vi "dfd_Lpth Norm Spec Convertion.vi"(8 "error in (no error)":errorcluster, 10 "filter specs":T2[](array[typedef]), 11 "order":i32=21) -> (0 "error out":errorcluster, 2 "band specification":T1 {"magnitude and weight"."frequency point"."weight" format="%.2f"}, 3 "order out":cluster{"# num":i32, "# den":i32}={"# num"=5, "# den"=5})   [LabVIEW 2017, in "NI_DigFilterLicensed.lvlib"]
uses:
  <vilib>/addons/Digital Filter Design/NI_DigFilterLicensed.lvlib
  <vilib>/addons/Digital Filter Design/_LpNorm.llb/dfd_Lp Norm Band Spec.ctl
  <vilib>/addons/Digital Filter Design/_Objects.llb/DFD Filter Specifiction (Design).ctl
panel:
  in  "band specification 2":T1 {"magnitude and weight"."frequency point"."weight" format="%.2f"}
  # "frequency"
  # "magnitude"
  # "weight"
  # "phase"
  # "frequency"
  # "magnitude"
  # "weight"
  # "phase"
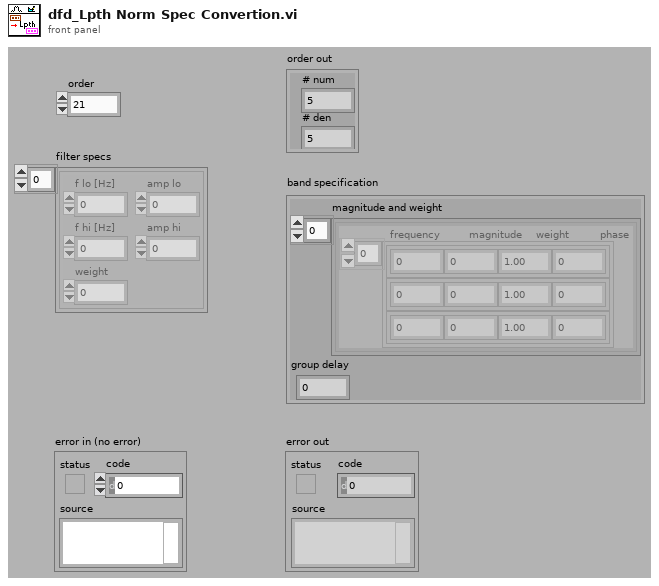
[diagram p1: front panel]
types:
  T1 = typedef "dfd_Lp Norm Band Spec.ctl" = cluster{"magnitude and weight":cluster{"frequency point":cluster{"frequency":dbl, "magnitude":dbl, "weight":dbl, "phase":dbl}[]}[], "group delay":dbl}
  T2 = typedef "NI_DigFilterLicensed.lvlib/DFD Filter Specifiction (Design).ctl" = cluster{"f lo [Hz]":dbl, "f hi [Hz]":dbl, "amp lo":dbl, "amp hi":dbl, "weight":dbl}
  T3 = cluster{"frequency point":cluster{"frequency":dbl, "magnitude":dbl, "weight":dbl, "phase":dbl}[]}[]
  T4 = cluster{"f lo [Hz]":dbl, "amp lo":dbl, "weight":dbl, dbl}
  T5 = cluster{"f hi [Hz]":dbl, "amp hi":dbl, "weight":dbl, dbl}
  T6 = cluster{"f hi [Hz]":dbl, "amp hi":dbl, "weight":dbl, dbl}[]
  T7 = cluster{"frequency point":cluster{"frequency":dbl, "magnitude":dbl, "weight":dbl, "phase":dbl}[]}
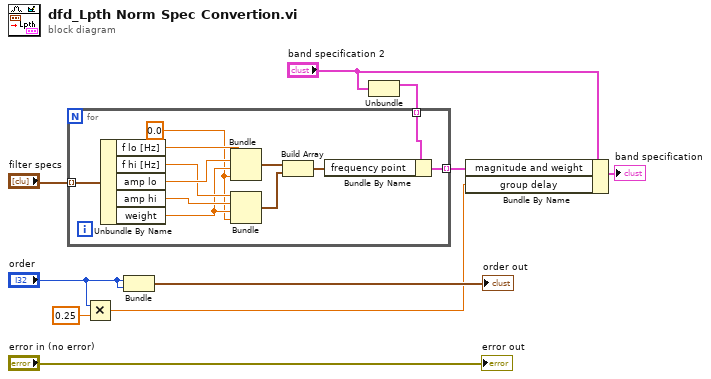
[diagram p0: block diagram]
diagram:
  n1 = Multiply(x="order", y=0.25) -> (x*y=w1:dbl)
  n2 = Bundle("order"="order", "order"="order") -> (→"order out":cluster{"order":i32, "order":i32})  [unwired: 1 out]
  n3 = Unbundle("band specification 2") -> ("magnitude and weight"=w4:T3)  [unwired: 1 out]
  n4 = for {
    tunnel: "filter specs" -> [w22] mode=indexing
    tunnel: w4 -> [w17] mode=indexing
    tunnel: [w15] -> w9 mode=indexing
    w11 = 0.0
    n5 = Unbundle By Name(w22) -> ("f lo [Hz]"=w14:dbl, "f hi [Hz]"=w13:dbl, "amp lo"=w21:dbl, "amp hi"=w20:dbl, "weight"=w12:dbl)
    n6 = Bundle("f lo [Hz]"=w14, "amp lo"=w21, "weight"=w12, w11) -> (w19:T4)  [unwired: 1 out]
    n7 = Bundle("f hi [Hz]"=w13, "amp hi"=w20, "weight"=w12, w11) -> (w18:T5)  [unwired: 1 out]
    n8 = Build Array(w19, w18) -> (w16:T6)
    n9 = Bundle By Name(cluster=w17, "frequency point"=w16) -> (w15:T7)
  }
  n10 = Bundle By Name(cluster="band specification 2", "magnitude and weight"=w9, "group delay"=w1) -> (→"band specification":T1)
  "error out" <- "error in (no error)"
